vi "DSComm.vi"(0 "Fire?":bool, 5 "Actual RPM":dbl, 7 "Desired RPM":dbl, 9 "Ball Pressure":dbl, 11 "error in (no error)":errorcluster) -> (15 "error out":errorcluster)   [LabVIEW 2011]
uses:
  Robot Global Data.vi
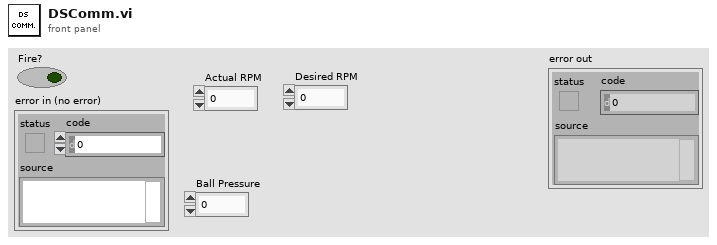
[diagram p1: front panel]
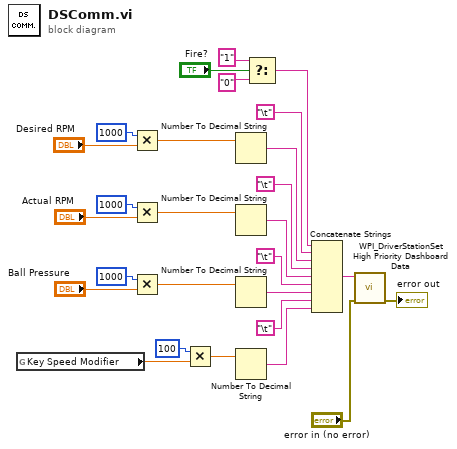
[diagram p0: block diagram]
diagram:
  n1 = global read "Robot Global Data.vi" "Key Speed Modifier"() -> (w2:dbl)
  n2 = Multiply(x=1000, y="Desired RPM") -> (x*y=w17:dbl)
  n3 = Multiply(x=1000, y="Actual RPM") -> (x*y=w14:dbl)
  n4 = Multiply(x=1000, y="Ball Pressure") -> (x*y=w8:dbl)
  n5 = Multiply(x=100, y=w2) -> (x*y=w3:dbl)
  n6 = Number To Decimal String(number=w17) -> (decimal integer string=w18:string)  [unwired: 1 in]
  n7 = Number To Decimal String(number=w14) -> (decimal integer string=w13:string)  [unwired: 1 in]
  n8 = Number To Decimal String(number=w8) -> (decimal integer string=w6:string)  [unwired: 1 in]
  n9 = Number To Decimal String(number=w3) -> (decimal integer string=w1:string)  [unwired: 1 in]
  n10 = Select(t="1", s="Fire?", f="0") -> (s? t:f=w25:string)
  n11 = Concatenate Strings(w25, "\t", w18, "\t", w13, "\t", w6, "\t", w1) -> (w24:string)
  n12 = call <vilib>:"WPI_DriverStationSet High Priority Dashboard Data.vi"("error in (no error)"="error in (no error)", "User Data"=w24) -> ("error out"=→"error out":errorcluster)  [unwired: 9 in]
